vi "convertFESTOtoBytes.vi"(8 "data":bool[](array[boolean]), 9 "Start Byte":i32, 11 "Bytes":u8[](array[numeric])) -> (3 "Bytes 2":u8[](array[numeric]))   [LabVIEW 2011]
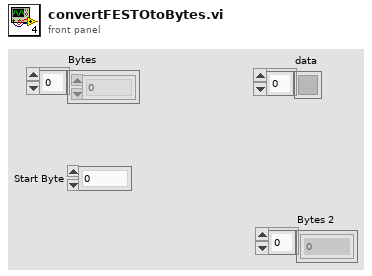
[diagram p1: front panel]
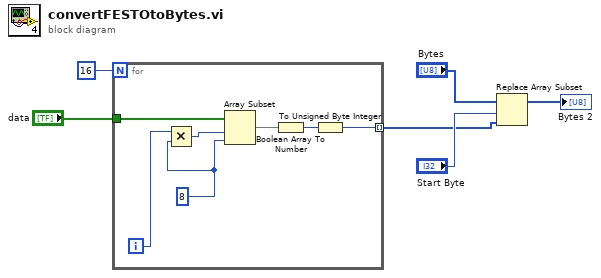
[diagram p0: block diagram]
diagram:
  n1 = for {
    N: 16 -> [_]
    tunnel: "data" -> [w13]
    tunnel: [w7] -> w2 mode=indexing
    i -> [w12]
    w11 = 8 ("length")
    n2 = Multiply(x=w12, y=w11) -> (x*y=w10:i32)
    n3 = Array Subset(array=w13, index=w10, length=w11) -> (w9:bool[])
    n4 = Boolean Array To Number(Boolean array=w9) -> (number=w8:u32)
    n5 = To Unsigned Byte Integer(number=w8) -> (unsigned 8bit integer=w7:u8)
  }
  n6 = Replace Array Subset(array="Bytes", new element=w2, index="Start Byte") -> (→"Bytes 2":u8[])
